vi "RM-read-error-code.vi"(8 "错误输入（无错误）":errorcluster, 11 "MB_Master_Serial输入":refnum<class "MB_Master_Serial.lvclass">) -> (0 "错误输出":errorcluster, 2 "error_code":i32, 3 "MB_Master_Serial输出":refnum<class "MB_Master_Serial.lvclass">)   [LabVIEW 2014]
uses:
  <vilib>/Plasmionique/MB Master/MB_Master_Serial/MB_Master_Serial.lvclass
  <vilib>/Plasmionique/MB Master/MB Master.lvlib
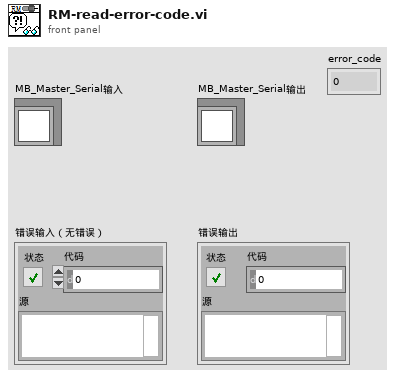
[diagram p1: front panel]
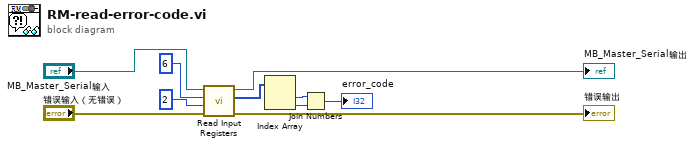
[diagram p0: block diagram]
diagram:
  n1 = call <vilib>:"Read Input Registers.vi"("error in (no error)"="错误输入（无错误）", "quantity"=u16 2, "starting address"=u16 6, "MB session in"="MB_Master_Serial输入") -> ("error out"=→"错误输出":errorcluster, "Registers"=w8:u16[], "MB session out"=→"MB_Master_Serial输出":refnum<class "MB_Master_Serial.lvclass">)  [unwired: 5 in]
  n2 = Index Array(array=w8) -> (element #1=w9:u16, element #2=w10:u16)  [unwired: 2 in]
  n3 = Join Numbers(hi=w9, lo=w10) -> ((hi.lo)=→"error_code":u32)
